vi "Alpha_Ver_1.1.vi"() -> ()   [LabVIEW 2015]
uses:
  <userlib>/LV-Link3/PolySubVIs/DtCreateAoutChan.vi
  <userlib>/LV-Link3/PolySubVIs/DtCreateAinChan.vi
  <userlib>/LV-Link3/PolySubVIs/DtOLReadMultipleSingle.vi
  <vilib>/addons/control/pid/pid.llb/PID (DBL).vi
  <userlib>/LV-Link3/PolySubVIs/DtOLWriteSingle.vi
  <vilib>/addons/control/pid/NI_PID_pid.lvlib
  <vilib>/ptbypt/NI_PtbyPt.lvlib
panel:
  in  "Adder":dbl(slide) scale=0.0..3.0
  in  "stop":bool
  in  "Input \nChannel":string="0"
  in  "Output \nChannel":string="0"
  in  "Device":string(combo)
  in  "PID gains":T1={"proportional gain (Kc)"=1.0, "integral time (Ti, min)"=0.01, "derivative time (Td, min)"=0.0} {"derivative time (Td, min)" format="%.3f"; "integral time (Ti, min)" format="%.3f"; "proportional gain (Kc)" format="%.3f"}
  in  "output range":cluster{"output high":dbl, "output low":dbl}={"output high"=10.0, "output low"=-10.0} {"output low" format="%.2f"; "output high" format="%.2f"}
  in  "Setpoint":dbl(slide) scale=0.0..10.0
  out "Meter":cluster{dbl, dbl}(knob)={0.0, 2.010068658273543} scale=0.0..10.0
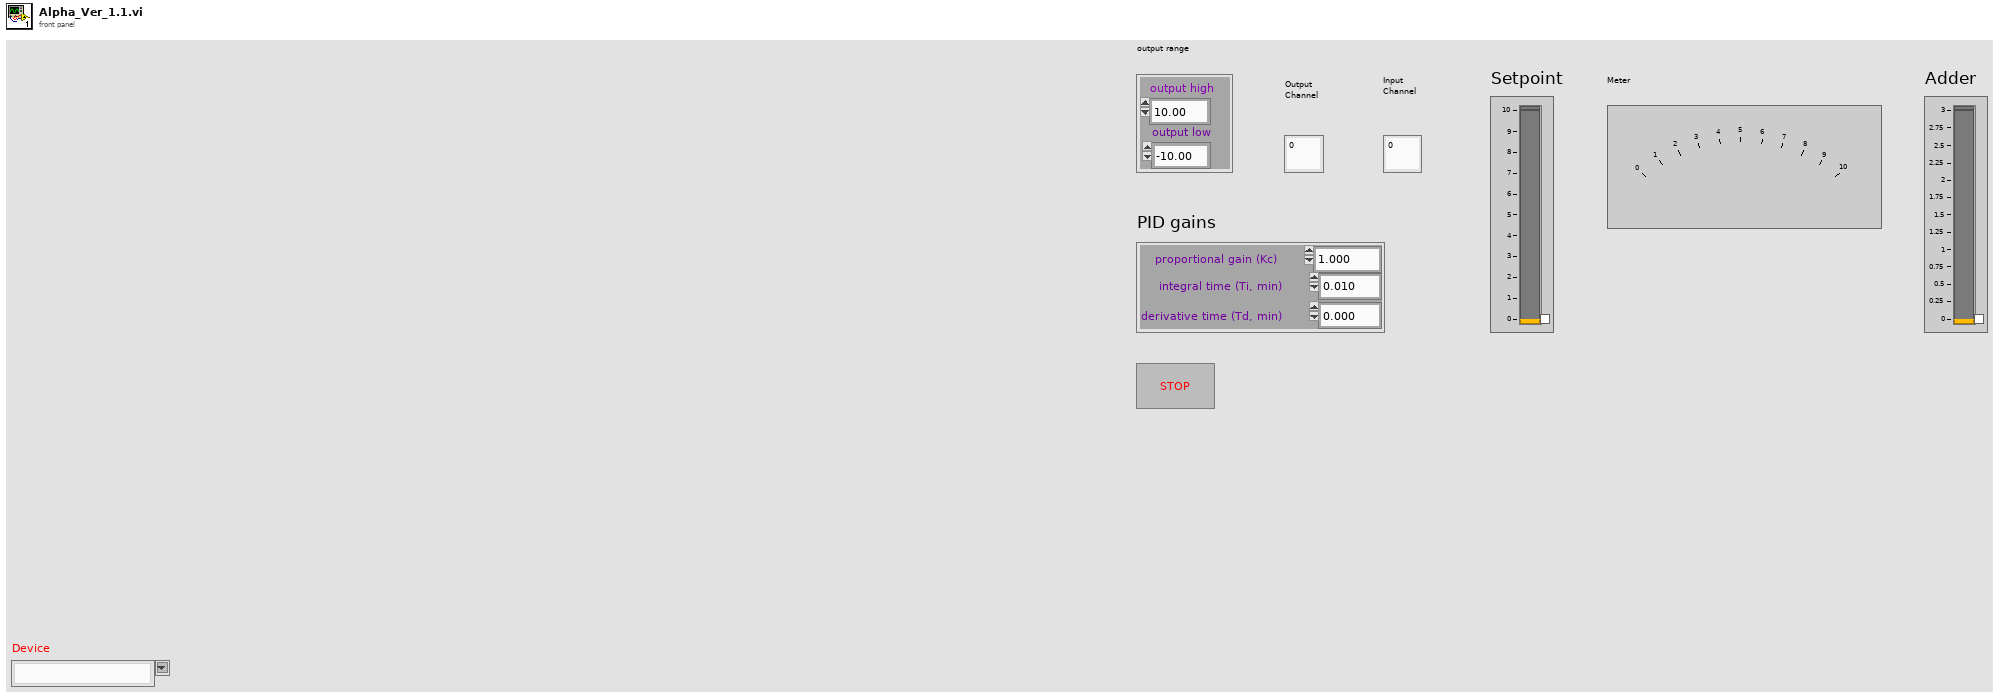
[diagram p1: front panel]
types:
  T1 = cluster{"proportional gain (Kc)":dbl, "integral time (Ti, min)":dbl, "derivative time (Td, min)":dbl}
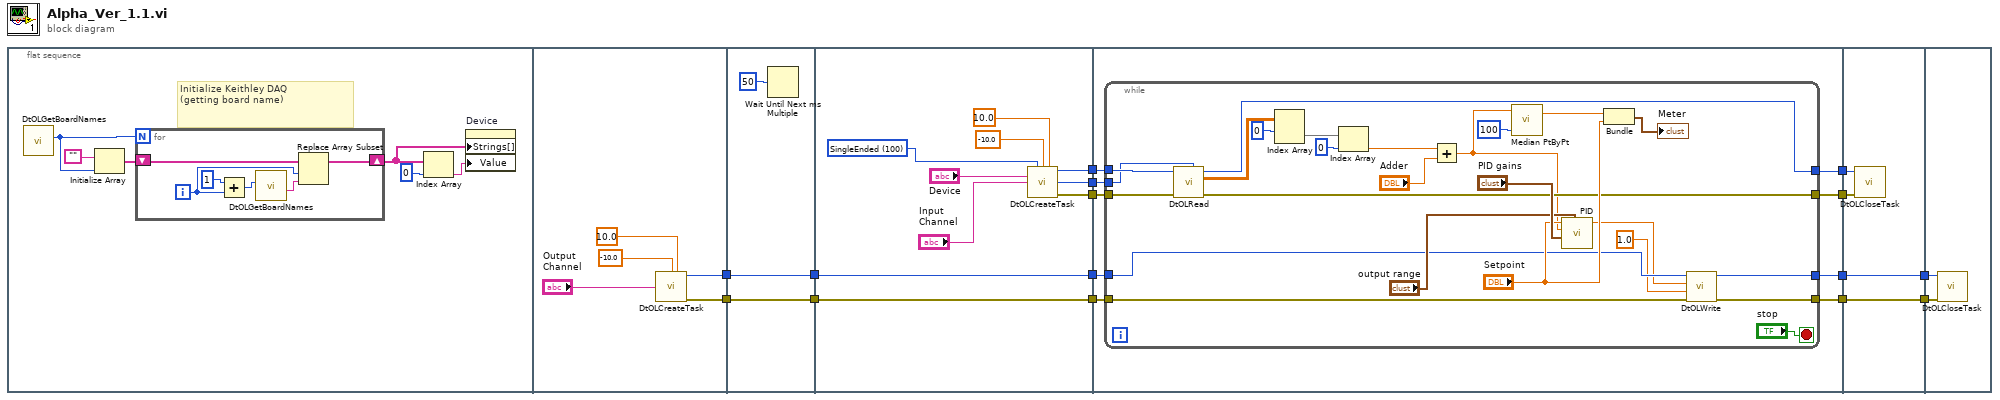
[diagram p0: block diagram]
diagram:
  n1 = flat-sequence {
    tunnel: [w28] -> w4
    tunnel: [w29] -> w2
    tunnel: w4 -> [w35]
    tunnel: [w35] -> w3
    tunnel: w2 -> [w34]
    tunnel: [w34] -> w1
    tunnel: [w41] -> w15
    tunnel: [w40] -> w14
    tunnel: [w39] -> w13
    tunnel: [w37] -> w12
    tunnel: [w36] -> w11
    tunnel: w3 -> [w36]
    tunnel: w1 -> [w37]
    tunnel: w15 -> [w54]
    tunnel: w14 -> [w53]
    tunnel: w13 -> [w52]
    tunnel: w12 -> [w51]
    tunnel: w11 -> [w50]
    tunnel: [w49] -> w10
    tunnel: [w48] -> w9
    tunnel: [w47] -> w8
    tunnel: [w46] -> w7
    tunnel: w10 -> [w81]
    tunnel: w9 -> [w80]
    tunnel: w8 -> [w83]
    tunnel: w7 -> [w82]
    tunnel: [w83] -> w6
    tunnel: [w82] -> w5
    tunnel: w6 -> [w85]
    tunnel: w5 -> [w84]
    frame #0 {
      # "Initialize Keithley DAQ \n(getting board name)"
      n2 = call <userlib>:"DtOLGetBoardNames.vi"() -> ("Number of boards"=w16:u32)  [unwired: 9 in, 2 out]
      n3 = Initialize Array("", w16) -> (w18:string[])
      n4 = for {
        N: w16 -> [_]
        shift-right: [w24] -> w21
        shift-left: w18 -> [w25]
        i -> [w23]
        n5 = Add(x=1, y=w23) -> (x+y=w27:i32)
        n6 = call <userlib>:"DtOLGetBoardNames.vi"("Select Board"=w27) -> ("Board Name"=w22:string)  [unwired: 8 in, 2 out]
        n7 = Replace Array Subset(array=w25, new element=w22, index=w23) -> (w24:string[])
      }
      n8 = Index Array(array=w21, index=0) -> (element=w20:string)
      n9 = property on="Device" class="CmbBox"("Strings[]"=w21, "Value"=w20) -> ()  [unwired: 2 in, 2 out]
    }
    frame #1 {
      n10 = call-poly <userlib>:"DtOLCreateTask.vi"("Range Min"=-10.0, "Range Max"=10.0, "Channel"="Output \nChannel") -> ("Task out"=w29:i32, "error out"=w28:errorcluster)  [unwired: 10 in, 1 out]
    }
    frame #2 {
      n11 = Wait Until Next ms Multiple(millisecond multiple=u32 50) -> ()  [unwired: 1 out]
    }
    frame #3 {
      w43 = 100 items=["SingleEnded"=100, "Differential"=101] ("Channel Type")
      n12 = call-poly <userlib>:"DtOLCreateTask.vi"("Channel Type"=w43, "Range Min"=-10.0, "Range Max"=10.0, "Board Name"="Device", "Channel"="Input \nChannel") -> ("Task out"=w41:i32, "Actual Number of Channels"=w40:u32, "error out"=w39:errorcluster)  [unwired: 8 in]
    }
    frame #4 {
      n13 = while {
        tunnel: w54 -> [w79]
        tunnel: w53 -> [w78]
        tunnel: w52 -> [w77]
        tunnel: w51 -> [w68]
        tunnel: w50 -> [w67]
        tunnel: [w63] -> w47
        tunnel: [w62] -> w46
        tunnel: [w61] -> w49
        tunnel: [w60] -> w48
        stop <- "stop" stop-if-true
        n14 = call-poly <userlib>:"DtOLRead.vi"("Number Chan to Read"=w78, "error in (no error)"=w77, "Task in"=w79) -> ("error out"=w60:errorcluster, "2D Data out"=w76:dbl[][], "Task out"=w61:i32)  [unwired: 4 in, 2 out]
        n15 = Index Array(array=w76, index (row)=0) -> (element=w74:dbl[])  [unwired: 1 in]
        n16 = Index Array(array=w74, index=0) -> (element=w56:dbl)
        n17 = Add(x=w56, y="Adder") -> (x+y=w55:dbl)
        n18 = call <vilib>:"Median PtByPt.vi"("sample length"=100, "x"=w55) -> ("median"=w58:dbl)  [unwired: 2 in, 1 out]
        n19 = call-poly <vilib>:"PID.vi"("output range"="output range", "PID gains"="PID gains", "process variable"=w55, "setpoint"="Setpoint") -> ("output"=w66:dbl)  [unwired: 6 in, 1 out]
        n20 = Bundle("median"=w58, "Setpoint"="Setpoint") -> (→"Meter":cluster{"median":dbl, "Setpoint":dbl})  [unwired: 1 in]
        n21 = call-poly <userlib>:"DtOLWrite.vi"("error in (no error)"=w67, "Timeout"=1.0, "Data In"=w66, "Task in"=w68) -> ("error out"=w62:errorcluster, "Task out"=w63:i32)  [unwired: 6 in]
      }
    }
    frame #5 {
      n22 = call <userlib>:"DtOLCloseTask.vi"("Error in"=w80, "Task in"=w81) -> ()  [unwired: 9 in, 1 out]
    }
    frame #6 {
      n23 = call <userlib>:"DtOLCloseTask.vi"("Error in"=w84, "Task in"=w85) -> ()  [unwired: 9 in, 1 out]
    }
  }
